vi "PvgeneratorOP500.vi"(8 "errin":errorcluster, 9 "BDD":T1, 10 "network":path, 11 "path in":path) -> (0 "sortie d'erreur":errorcluster caption="errout", 1 "network out":path, 2 "tout bon":bool, 3 "Chaîne":string)   [LabVIEW 2020]
uses:
  VG/IS30%.vi
  VG/PN.vi
panel:
  out "PDU+":string
  out "PDU-":string
  out "Tab1":string[][](array[string])
  out "nombre de remplacements":i32
  # "16/10/2023_08:15:59"
  # "2023-10-04 15:58:32"
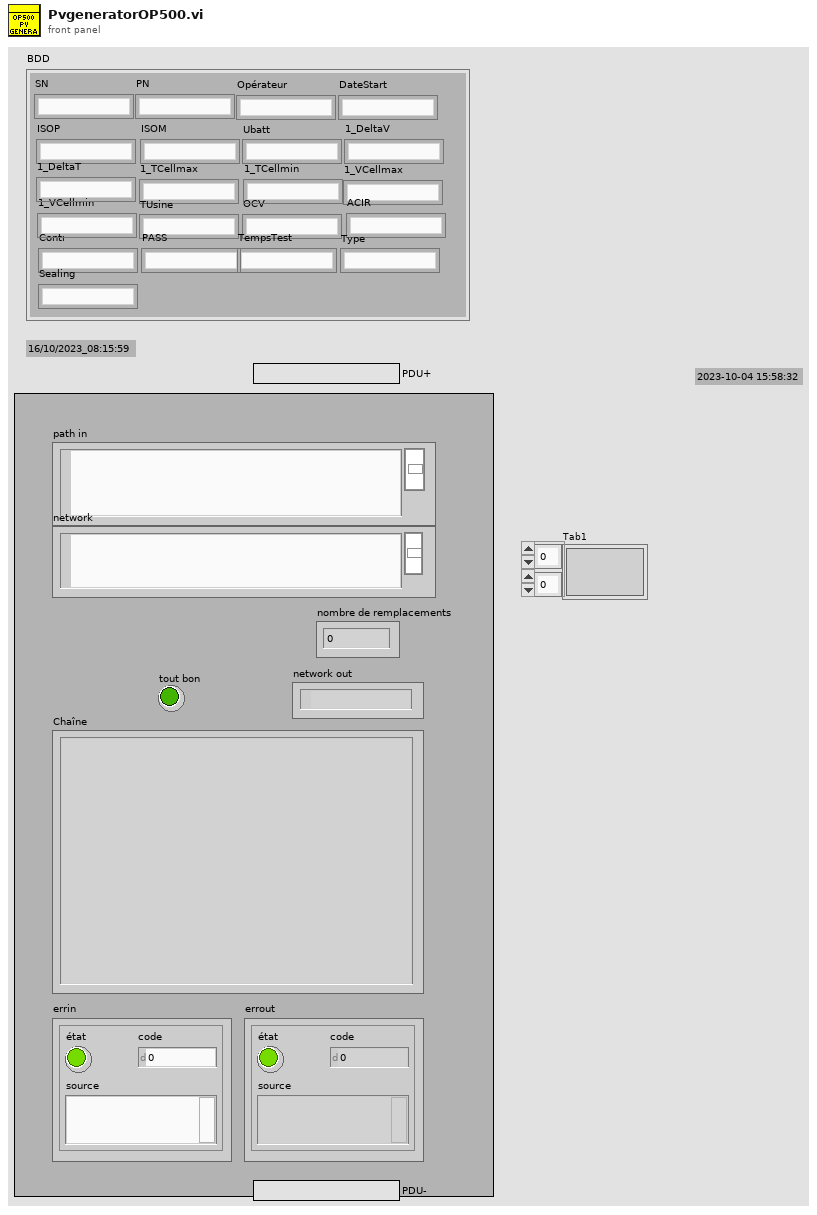
[diagram p1: front panel]
types:
  T1 = cluster{"SN":string, "PN":string, "Opérateur":string, "DateStart":string, "ISOP":string, "ISOM":string, "Ubatt":string, "1_DeltaV":string, "1_DeltaT":string, "1_TCellmax":string, "1_TCellmin":string, "1_VCellmax":string, "1_VCellmin":string, "TUsine":string, "OCV":string, "ACIR":string, "Conti":string, "PASS":string, "TempsTest":string, "Type":string, "Sealing":string}
  T2 = enum16{"open", "replace", "create", "open or create", "replace or create", "replace or create with confirmation"}
  T3 = cluster{string, string, string, string, string, string, string, string, string, string}
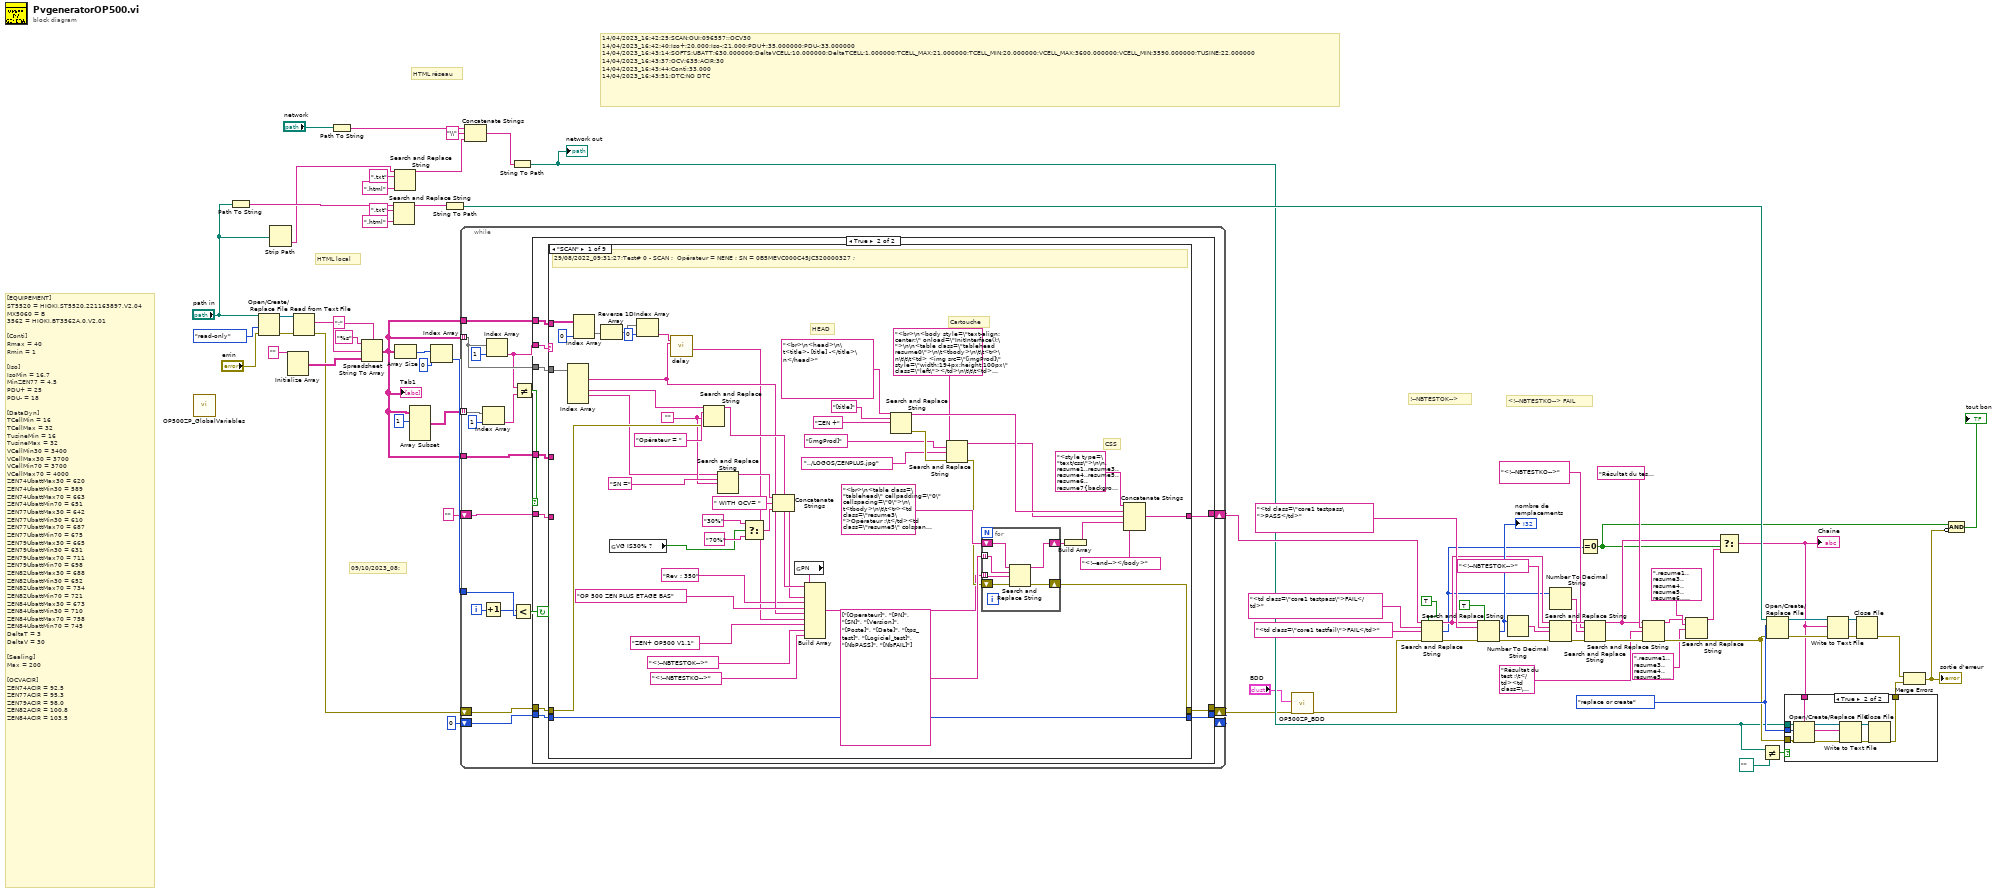
[diagram p0: block diagram]
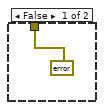
[diagram p2: hidden frame]
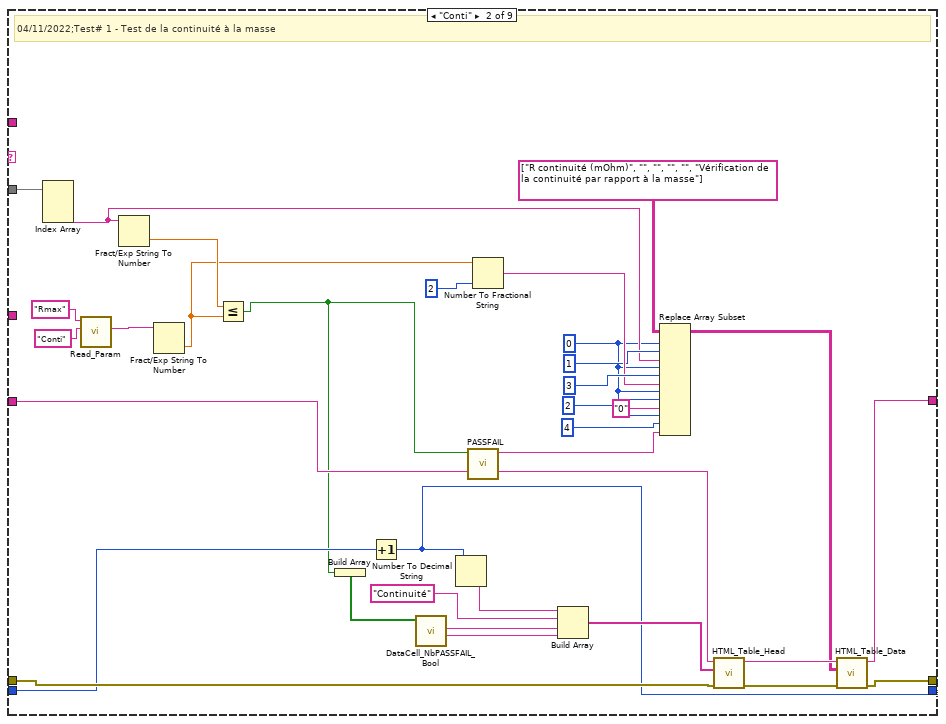
[diagram p4: hidden frame]
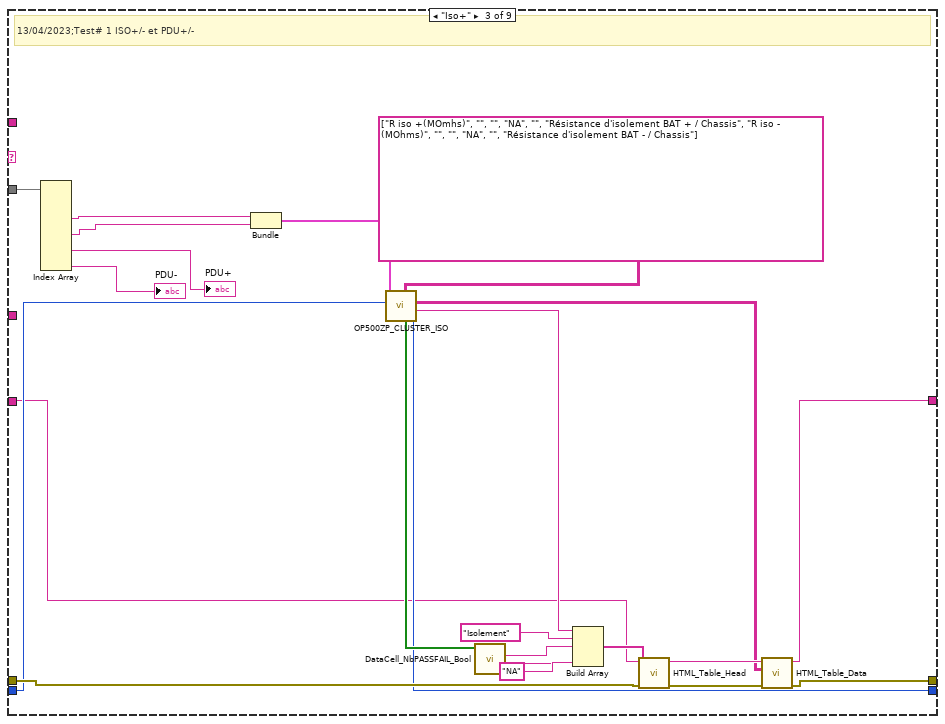
[diagram p5: hidden frame]
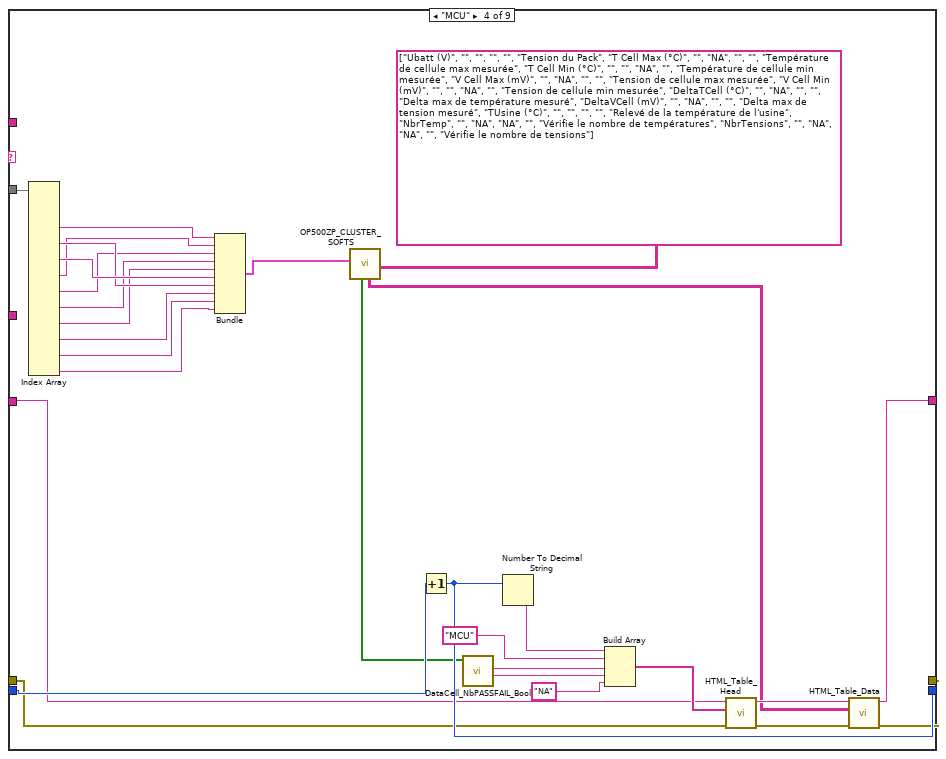
[diagram p6: hidden frame]
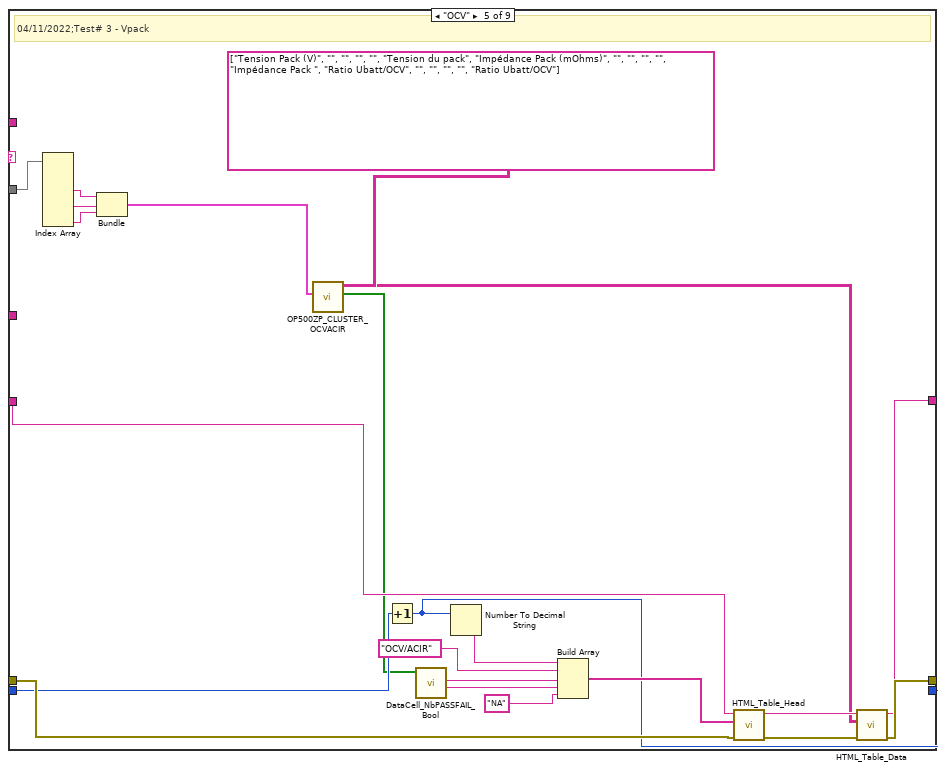
[diagram p7: hidden frame]
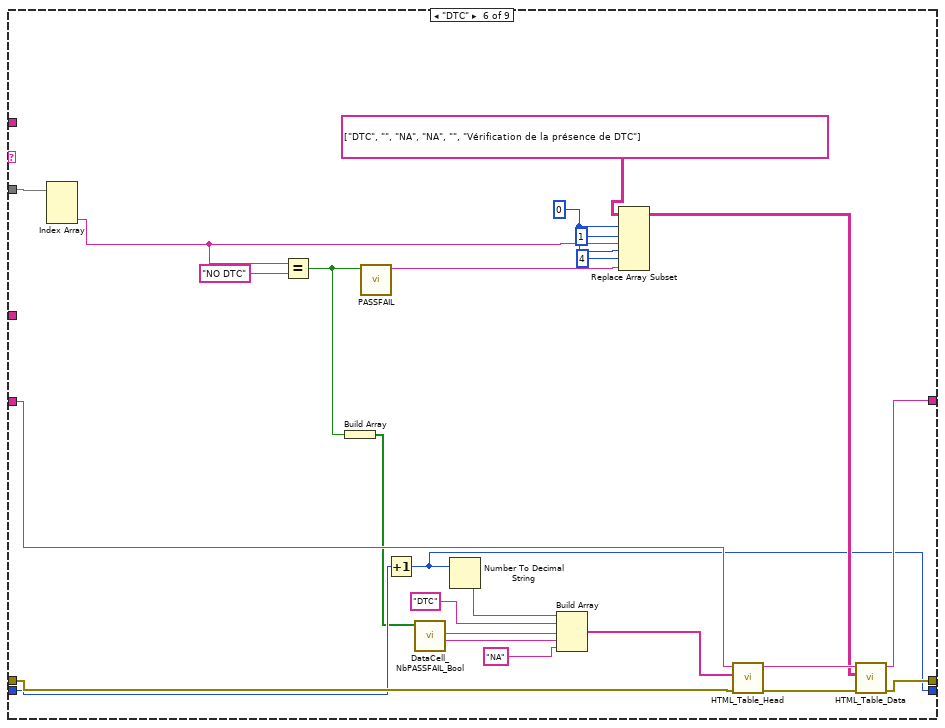
[diagram p8: hidden frame]
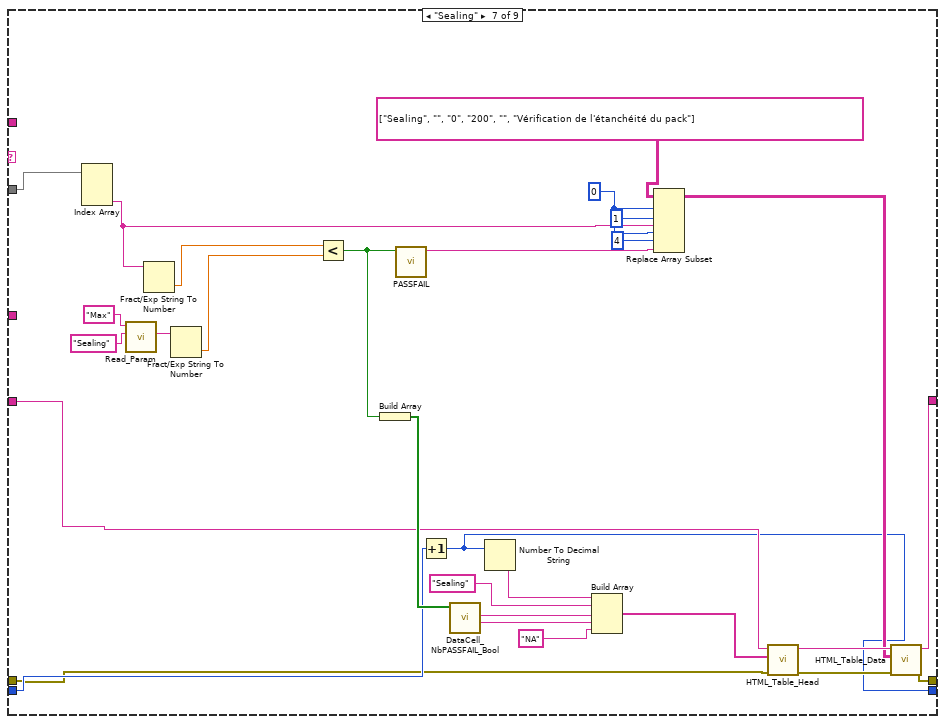
[diagram p9: hidden frame]
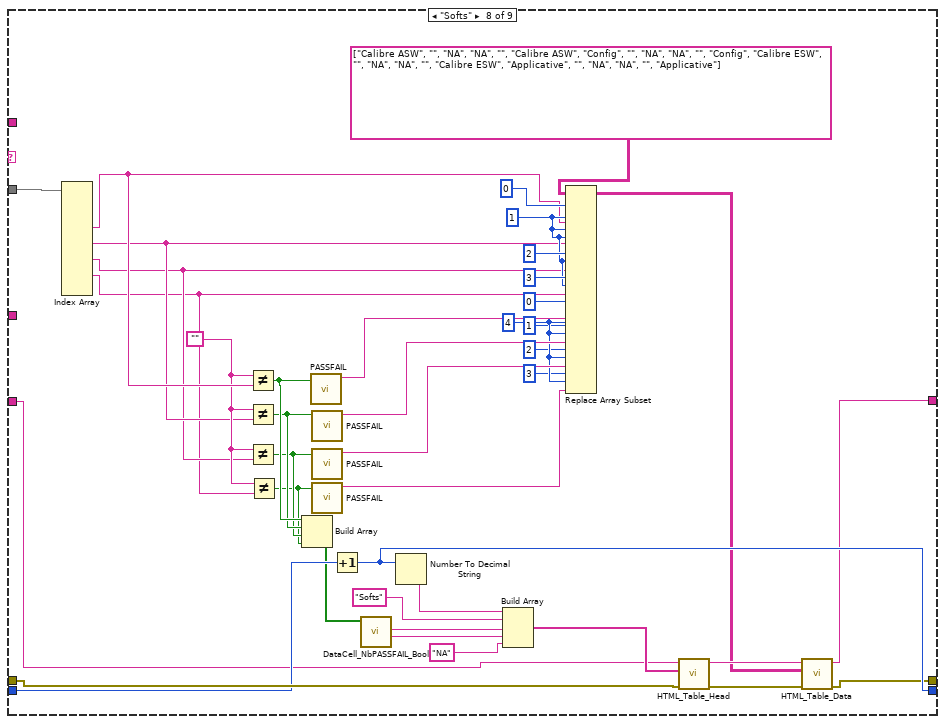
[diagram p10: hidden frame]
diagram:
  w36 = T2."replace or create" ("opération (0 : open)")
  # "09/10/2023_08:"
  # "HTML réseau"
  # "HTML local"
  # "14/04/2023_16:42:25;SCAN;OUI;096557;;OCV30\n14/04/2023_16:42:40;Iso+;20,000;Iso-;21,000;PDU+;35,000000;PDU-;33,000000\n14/04/2023_16:43:14;SOFTS;UBATT;630,000000;DeltaVCELL;10,000000;DeltaTCELL;1,000000;TCELL_MAX;21,000000;TCELL_MIN;20,000000;VCELL_MAX;3600,000000;VCELL_MIN;3590,000000;TUSINE;22,000000\n14/04/2023_16:43:37;OCV;635;ACIR;30\n14/04/2023_16:43:44;Conti;33,000\n14/04/2023_16:43:51;DTC;NO DTC"
  # "[EQUIPEMENT]\nST5520 = HIOKI,ST5520,221163897,V2.04\t\nMX5060 = B\n3562 = HIOKI,BT3562A,0,V2.01\n\n[Conti]\nRmax = 40\nRmin = 1\n\n[Iso]\nIsoMin = 16.7\nMinZEN77 = 4.5\nPDU+ = 25\nPDU- = 18\n\n[DataDyn]\nTCellMin = 16\nTCellMax = 32\nTusineMin = 16\nTusineMax = 32\nVCellMin30 = 3400\nVCellMax30 = 3700\nVCellMin70 = 3700\nVCellMax70 = 4000\nZEN74UbattMax30 = 620\nZEN74UbattMin30 = 589\nZEN74UbattMax70 = 663\nZEN74UbattMin70 = 651\nZEN77UbattMax30 = 642\nZEN77UbattMin30 = 610\nZEN77UbattMax70 = 687\nZEN77UbattMin70 = 675\nZEN79UbattMax30 = 665\nZEN79UbattMin30 = 631\nZEN79UbattMax70 = 711\nZEN79UbattMin70 = 698\nZEN82UbattMax30 = 688\nZEN82UbattMin30 = 652\nZEN82UbattMax70 = 734\nZEN82UbattMin70 = 721\nZEN84UbattMax30 = 673\nZEN84UbattMin30 = 710\nZEN84UbattMax70 = 758\nZEN84UbattMin70 = 745\nDeltaT = 3\nDeltaV = 30\n\n[Sealing]\nMax = 200\n\n[OCVACIR]\nZEN74ACIR = 92.5\nZEN77ACIR = 95.3\nZEN79ACIR = 98.0\nZEN82ACIR = 100.8\nZEN84ACIR = 103.5"
  # "<!--NBTESTKO--> FAIL"
  # "!--NBTESTOK-->"
  n1 = call "OP500ZP_GlobalVariables.vi"() -> ()  [unwired: 12 in]
  n2 = Path To String(path="path in") -> (string=w57:string)
  n3 = Open/Create/Replace File(file path (use dialog)="path in", error in="errin", access (0:read/write)=enum16{"read/write", "read-only", "write-only"}."read-only" ("accès (0 : read/write)")) -> (refnum out=w58:refnum<file>, error out=w74:errorcluster)  [unwired: 3 in, 1 out]
  n4 = Strip Path(path="path in") -> (name=w17:string)  [unwired: 1 out]
  n5 = Initialize Array("") -> (w72:string[][])  [unwired: 2 in]
  n6 = Read from Text File(file (use dialog)=w58, error in=w74) -> (text=w70:string, error out=w4:errorcluster)  [unwired: 2 in, 2 out]
  n7 = Path To String(path="network") -> (string=w16:string)
  n8 = Spreadsheet String To Array(delimiter (Tab)=";" ("séparateur (Tabulation)"), format string="%s" ("chaîne de format"), spreadsheet string=w70, array type (2D Dbl)=w72) -> (array=w7:string[][])
  "Tab1" <- w7
  n9 = Search and Replace String(input string=w57, search string=".txt" ("chaîne recherchée"), replace string=".html" ("chaîne de remplacement (\"\")")) -> (result string=w54:string)  [unwired: 5 in, 3 out]
  n10 = Search and Replace String(input string=w17, search string=".txt" ("chaîne recherchée"), replace string=".html" ("chaîne de remplacement (\"\")")) -> (result string=w14:string)  [unwired: 5 in, 3 out]
  n11 = Array Size(array=w7) -> (size(s)=w68:i32[])
  n12 = Array Subset(array=w7, index (row)=1 ("indice")) -> (w5:string[][])  [unwired: 3 in]
  n13 = Index Array(array=w68, index=0 ("indice")) -> (element=w66:i32)
  n14 = String To Path(string=w54) -> (path=w53:path)
  n15 = while {
    tunnel: w66 -> [w93]
    tunnel: w7 -> [w90] mode=indexing
    shift-right: [w89] -> w1
    shift-left: w4 -> [w88]
    shift-right: [w82] -> w52
    shift-left: "" -> [w87]
    shift-right: [w85] -> _
    shift-left: 0 -> [w86]
    tunnel: w7 -> [w84]
    tunnel: w7 -> [w81]
    tunnel: w5 -> [w79] mode=indexing
    i -> [w94]
    stop <- w92 continue-if-true
    n16 = Index Array(array=w79, index=1 ("indice")) -> (element=w78:string)
    n17 = Increment(x=w94) -> (x+1=w83:i32)
    n18 = Index Array(array=w90, index=1 ("indice")) -> (element=w77:string)
    n19 = Less?(x=w83, y=w93) -> (x < y?=w92:bool)
    n20 = Not Equal?(x=w77, y=w78) -> (x != y?=w76:bool)
    n21 = case shown="True" w76 {
      tunnel: w90 -> [_ w107]
      tunnel: [w96 w106] -> w89
      tunnel: w88 -> [w96 w105]
      tunnel: w87 -> [w97 w104]
      tunnel: w86 -> [w95 w103]
      tunnel: [w95 w102] -> w85
      tunnel: w84 -> [_ w101]
      tunnel: [w97 w100] -> w82
      tunnel: w77 -> [_ w99]
      tunnel: w81 -> [_ w98]
      frame False {
      }
      frame True {
        n22 = case shown="\"SCAN\"" w99 {
          tunnel: w105 -> [w154 w188 w211 w235 w261 w286 w305 w335 w366]
          tunnel: w107 -> [w156 w189 w212 w247 w262 w279 w307 w363 _]
          tunnel: [w133 w187 w210 w233 w260 w285 w302 w327 w366] -> w106
          tunnel: w104 -> [_ w186 w202 w232 w259 w280 w304 w324 w364]
          tunnel: w103 -> [w132 w185 w209 w239 w258 w284 w306 w334 w365]
          tunnel: [w132 w184 w203 w238 w257 w270 w301 w333 w365] -> w102
          tunnel: w101 -> [_ _ _ _ _ _ _ _ _]
          tunnel: [w131 w183 w208 w237 w256 w281 w303 w326 w364] -> w100
          tunnel: w98 -> [w110 _ _ _ _ _ _ _ _]
          frame "SCAN" {
            w127 = ""
            # "Cartouche"
            # "HEAD"
            # "CSS"
            # "29/08/2022_09:31:27;Test# 0 - SCAN ;  Opérateur = NENE ; SN = 0B5MEVC000C45JC320000327 ;"
            n23 = Index Array(array=w156) -> (element #1=w125:string, element #3=w130:string, element #4=w126:string)  [unwired: 5 in, 2 out]
            n24 = Index Array(array=w110, index (col)=0 ("disabled index (col)")) -> (element=w113:string[])  [unwired: 1 in]
            n25 = Reverse 1D Array(array=w113) -> (reversed array=w112:string[])
            n26 = global read "IS30%.vi" "VG IS30% ?"() -> (w117:bool)
            n27 = Index Array(array=w112, index=0) -> (element=w109:string)
            n28 = call "delay.vi"("String"=w125, "String 2"=w109) -> ("Delay calculé"=w108:string)  [unwired: 9 in]
            n29 = Search and Replace String(input string=w130, search string="Opérateur = " ("chaîne recherchée"), replace string=w127, error in=w154) -> (result string=w129:string)  [unwired: 4 in, 3 out]
            n30 = Search and Replace String(input string=w126, search string="SN =" ("chaîne recherchée"), replace string=w127) -> (result string=w123:string)  [unwired: 5 in, 3 out]
            n31 = Select(t="30%" ("y"), s=w117, f="70%" ("y")) -> (s? t:f=w120:string)
            n32 = Concatenate Strings(w123, " WITH OCV= " ("chaîne"), w120) -> (w122:string)
            n33 = global read "PN.vi" "PN"() -> (w116:string)
            n34 = Build Array(w129, w116, w122, "Rev : 350" ("élément"), "OP 500 ZEN PLUS ETAGE BAS" ("chaîne"), w125, w108, "ZEN+ OP500 V1.1" ("chaîne"), "<!--NBTESTOK-->" ("chaîne"), "<!--NBTESTKO-->" ("chaîne")) -> (w134:string[])
            n35 = Search and Replace String(input string="<br>\n<head>\n\t<title>- [title] -</title>\n</head>", search string="[title]" ("chaîne recherchée"), replace string="ZEN +" ("Title")) -> (result string=w150:string, error out=w149:errorcluster)  [unwired: 5 in, 2 out]
            n36 = Search and Replace String(input string="<br>\n<body style=\"text-align: center;\" onload=\"InitInterface();\">\n\n<table class=\"tablehead resume0\">\n\t<tbody>\n\t\t<tr>\n\t\t\t<td> <img src=\"[imgProd]\" style=\"width:194px;height:100px\" class=\"left\"></td>\n\t\t\t<td> <div class=\"center\">PROCES VERBAL DE TEST AUTOMATIQUE</div><div class=\"center\">Zen Plus OP 500</div><br class=\"center\"><div class=\"center\">Forseepower</div></td>\n\t\t\t<td> <img src=\"../LOGOS/LOGO FORSEE.png\" style=\"width:194px\"  class=\"right\"></td>\n\t\t</tr>\n\t</tbody>\n</table>", search string="[imgProd]", replace string="../LOGOS/ZENPLUS.jpg" ("imgProd"), error in=w149) -> (result string=w147:string, error out=w144:errorcluster)  [unwired: 4 in, 2 out]
            n37 = for {
              shift-right: [w161] -> w143
              shift-left: "<br>\n<table class=\"tablehead\" cellpadding=\"0\" cellspacing=\"0\">\n\t<tbody>\n\t\t<tr><td class=\"resume3\">Opérateur :\t</td><td class=\"resume5\" colspan=\"3\">[Operateur]</td></tr>\n\t\t<tr><td class=\"resume3\">PN : </td><td class=\"resume5\" colspan=\"3\">[PN]</td></tr>\n\t\t<tr><td class=\"resume3\">SN : </td><td class=\"resume5\" colspan=\"3\">[SN]</td></tr>\n\t\t<tr><td class=\"resume3\">Version : </td><td class=\"resume5\" colspan=\"3\">[Version]</td></tr>\n\t\t<tr><td class=\"resume3\">Poste : </td><td class=\"resume5\" colspan=\"3\">[Poste]</td></tr>\t\t\n\t\t<tr><td class=\"resume3\">Date du test : </td><td class=\"resume5\" colspan=\"3\">[Date]</td></tr>\n\t\t<tr><td class=\"resume3\">Temps de test : </td><td class=\"resume5\" colspan=\"3\">[tps_test]</td></tr>\n\t\t<tr><td class=\"resume3\">Logiciel de test :\t</td><td class=\"resume5\" colspan=\"3\">[Logiciel_test]</td></tr>\n\t\t<tr><td class=\"resume3\">Résultat du test :\t</td><td class=\"resume5\" colspan=\"3\"><div><span style=\"float:left\" id=\"result\"><font size = \"5pt\" color=\"green\"><b>CONFORME</b></font><b><font size = \"5pt\"> ( </font><font size = \"5pt\" color=\"green\">[NbPASS] PASS </font>  <font size = \"5pt\"> / </font><font size = \"5pt\" color=\"red\">[NbFAIL] FAIL</font> <font size = \"5pt\"> ) </font></b></span></div></td></tr>\n\t</tbody>\n</table>" -> [w162]
              tunnel: string[] ["[Operateur]", "[PN]", "[SN]", "[Version]", "[Poste]", "[Date]", "[tps_test]", "[Logiciel_test]", "[NbPASS]", "[NbFAIL]"] -> [w158] mode=indexing
              tunnel: w134 -> [w157] mode=indexing
              shift-right: [w159] -> w133
              shift-left: w144 -> [w160]
              n38 = Search and Replace String(input string=w162, search string=w158, replace string=w157, error in=w160) -> (result string=w161:string, error out=w159:errorcluster)  [unwired: 4 in, 2 out]
            }
            n39 = Build Array(w143) -> (w142:string[])
            n40 = Concatenate Strings("<style type=\"text/css\">\n\n.resume1,.resume3,.resume4,.resume5,.resume6,.resume7{background-color:#e6feef;padding:7px;border:1px solid black;}\n.resume0{border:1px solid black;background-color:#e6feef;font-weight: bold;padding:0px;text-align: center;}\n.resume1{width:350px;text-align:right;font-weight:bold;}\n.resume3{width:350px;text-align:right;border-top:0px solid black;font-weight:bold;}\n.resume4{border-left:0px solid black;width:290px;}\n.resume5{width:290px;border-left:0px solid black;border-top:0px solid black;}\n.resume6{border-left:0px solid black;width:60px;}\n.resume7{border-left:0px solid black;border-top:0px solid black;width:60px;}\n.title1{text-align: left;background-color:#e6f4fe;padding:10px;border:1px solid #101010;}\n.title2{width: 30px;text-align: center;background-color:#e6f4fe;padding:1px;border:1px solid #101010;border-left:0px solid black;font-weight: bold;}\n.title2 a:link{text-decoration:none;}\n.entete0,.entete1,.entete2,.time2{text-align: center;background-color:#feeec9;padding:7px;border:1px solid black;font-weight: bold;}\n.entete0{width:45px;border-right:0px solid black;}\n.entete1{width:505px;}\n.entete2{width:95px;border-right:0px solid black;}\n.time2{border-left:0px solid black;width:145px;font-size:11px;}\n.core0,.core1,.core2,.core3,.core4,.time{text-align: center;background-color:#fafed3;padding:7px;border:1px solid black;}\n.core0, .core1,.core3,.core4{width:95px;border-top:0px solid black;border-right:0px solid black;}\n.core0{width:45px;}\n.core2{border-top:0px solid black;width:505px;}\n.core3{width:200px;}\n.core4{width:300px;}\n.time{width:145px;border-top:0px solid black;border-left:0px solid black;font-size:11px;}\n.false .core0,.false .core1,.false .core2,.false .core3,.false .core4,.false .time{background-color:#f4f4f4;}\n.false .entete0,.false .entete1,.false .entete2,.false .time2{background-color:#dadada;}\n.false .title1,.false .title2,.false .resultentete .testpass,.false .resultentete .testfail,.false .resultentete .testtime{background-color:#c5cac9;color: blue;}\n.false .title2 a:link{text-decoration:none;color: blue;}\n.comment1,.comment2,.time3{width: 890px;background-color:#e9e8e9;padding:7px;border:1px solid black;border-top:0px solid black;text-align:left;}\n.comment2{border-right:0px solid black;width: 45px;text-align: center;}\n.time3{width: 145px;border-left:0px solid black;font-size:11px;}\n.fixe1{background: -moz-linear-gradient(center top , #101010 10%, #555555 80%) repeat scroll 0 0 transparent;background: -webkit-gradient(linear, left top, left bottom, from(#101010), to(#555555));border:2px solid orange;position : fixed;margin-top:20px;display:none;overflow-y:scroll;max-height:350px;text-shadow: 0px 0px 0 #333333;text-align:left;font-size:10px;padding:10px;margin-left:-162px;border-radius: 15px 15px 15px 15px;}\n.menufixe, .menufixelock{background: -moz-linear-gradient(center top , #101010 80%, transparent 20%) repeat scroll 0 0 transparent;background: -webkit-gradient(linear, left top, left bottom, from(#101010), color-stop(0.65, #101010), to(transparent)) repeat scroll 0 0 transparent;margin: -52px 0px 0px -9px;width:100%;position:fixed;height:55px;-moz-transition: margin 1s;-webkit-transition: margin 1s;}\n.menufixelock, .menufixe:hover{margin: -9px 0px 0px -9px;}\n.lockmenu, .separation,.separationmenu{text-align:center;background: -moz-linear-gradient(center top , #555555 10%, #111111 80%) repeat scroll 0 0 transparent;background: -webkit-gradient(linear, left top, left bottom, from(#555555), to(#111111));border: 1px solid white;border-radius: 10px 10px 10px 10px;box-shadow: 0 -1px 1px #555555 inset;color: #999999;font-weight: bold;width: 100px;padding: 2px;text-decoration: none;}\n.tablehead{width: 1000px;font-family: Verdana;font-size: 12px;margin-left: auto;margin-right: auto;}\n.tablenull{font-family: Verdana;font-size: 11px;margin-left: auto;margin-right: auto;}\n.separationmenu:hover div{display: inline;}\n.lockmenu:hover, .separation:hover,.separationmenu:hover{border: 1px solid orange;cursor:pointer;}\n.lockmenu:hover{border: 1px solid red;cursor:pointer;}\n.separationright{padding:10px;}\ndiv a:link{text-decoration:none;color:#cbcbcb;}\ndiv a:hover{text-decoration:underline;color:#cbcbcb;}\nspan a:link{text-decoration:none;color:#cbcbcb;}\nspan a:hover{text-decoration:none;color:#cbcbcb;}\n.false{color: blue;}\n.testpass{color: green;font-weight: bold;}\n.testfail{color: red;font-weight: bold;}\n.testtime{color: blue;font-weight: bold;}\n.resultentete{font-weight: bold;font-size: 11px;min-width: 200px;text-align:right;}\n.infohard{border: 1px solid black;background-color: white;text-align: center;width: 16px;height: 16px;border-radius: 5px;font-weight: bold;box-shadow: 0 -1px 2px #555555 inset;}\n.infohard:hover{background-color:#feeec9;cursor:pointer;}\n.footerhard{padding-top:30px;}\n.confighard{font-size:10px;width:110px;}\n.circlemain{margin-left:auto;margin-right:auto;}\n.circletext,.circleform{padding-top: 3px;text-align:center;font-size: 10px;width:200px;}\n.circleform{padding-bottom: 3px;padding-top: 1px;}\n.circle{border: 1px solid black;border-collapse: collapse;border-radius: 15px;box-shadow: 1px 1px 0 #505050;height: 15px;width: 15px;display:inline-block;}\n.bookmarkon, .bookmarkoff{background-color: yellow;border: 1px solid black;border-collapse: collapse;border-radius: 10px 10px 10px 10px;box-shadow: 1px 1px 0 #505050;height: 12px;width: 12px;position: absolute;margin-left:22px;cursor: help;}\n.bookmarkoff{background-color: transparent;border: 1px solid #CECECE;box-shadow: none;cursor: copy;}\n.false .bookmarkoff{background-color: transparent;border: 1px solid #E6E1E1;box-shadow: none;cursor: copy;}\n.bookmarkmaster{height: 15px;margin-right: 12px;width: 60px;}\n.bookmarkmaster:hover .bookmarkprev,.bookmarkmaster:hover .bookmarksuiv{display:block;}\n.bookmarkprev, .bookmarksuiv {cursor: pointer;font-size: 25px;font-weight: bold;margin-top: -10px;position: absolute;display:none;}\n.bookmarkprev{margin-left: 2px;}\n.bookmarksuiv{margin-left: 43px;}\n.plus, .moins{background-color: #F4F4F4;border: 1px solid #848484;border-radius: 20px;color: #848484;font-family: arial;font-size: 16px;font-weight: bold;height: 20px;margin-left: 4px;text-align: center;width: 20px;}\n.moins{font-size: 15px;}\n.plus:hover, .moins:hover{background-color: #DADADA;border: 1px solid black;color: black;cursor:pointer;}\n.backtothetop {position: fixed; right: 50%; margin-right: -555px; bottom: 10px; font-size: 35px; font-weight: bold; border: 1px solid #7D7B91; width: 40px; height: 40px; line-height:52px; text-align: center;border-radius: 8px; opacity: 0.25; background-color: #F5F5F5; color:#7D7B91;}\n.backtothetop:hover {opacity: 1; cursor:pointer;}\n.libversion {font-size: 8px;font-weight: normal;padding-right: 10px;text-align: right;}\n.lockmenu {width: 18px;font-size: 12px;}\n.left {display: block; margin-left: 1px;margin-right: auto;}\n.right {display: block; margin-right: 1px;margin-left: auto;}\n.center {display: block; margin-left: auto;margin-right: auto;}\n\n</style>", w150, w147, w142, "<!--end--></body>") -> (w131:string)
          }
          frame "Conti" {
            w171 = 0 ("index (row)")
            # "04/11/2022;Test# 1 - Test de la continuité à la masse"
            n41 = Index Array(array=w189) -> (element #3=w174:string)  [unwired: 3 in, 2 out]
            n42 = call <userlib>:"Read_Param.vi"("section"="Conti", "key"="Rmax") -> ("str"=w166:string)  [unwired: 5 in, 4 out]
            n43 = Fract/Exp String To Number(string=w174) -> (number=w169:dbl)  [unwired: 3 in, 1 out]
            n44 = Fract/Exp String To Number(string=w166) -> (number=w163:dbl)  [unwired: 3 in, 1 out]
            n45 = Less Or Equal?(x=w169, y=w163) -> (x <= y?=w168:bool)
            n46 = Build Array(w168) -> (w181:bool[])
            n47 = Increment(x=w185) -> (x+1=w184:i32)
            n48 = call <userlib>:"DataCell_NbPASSFAIL_Bool.vi"("Tableau en entrée"=w181) -> ("Chaîne"=w179:string, "Chaîne 2"=w180:string)  [unwired: 8 in, 1 out]
            n49 = Number To Decimal String(number=w184) -> (decimal integer string=w191:string)  [unwired: 1 in]
            n50 = call <userlib>:"PASSFAIL.vi"("E"=w168) -> ("S"=w173:string)  [unwired: 10 in]
            n51 = Number To Fractional String(number=w163, precision (6)=i16 2) -> (F-format string=w177:string)  [unwired: 2 in]
            n52 = Build Array(w191, "Continuité" ("élément"), w180, w179) -> (w194:string[])
            n53 = Replace Array Subset(array=string[][] [["R continuité (mOhm)", "", "", "", "", "Vérification de la continuité par rapport à la masse"]] ("Tableau"), new element #1=w174, index (row) #1=w171, index (col) #1=1 ("disabled index (col)"), new element #2=w177, index (row) #2=w171, index (col) #2=3 ("disabled index (col)"), new element #3="0" ("nouvel élément/sous-tableau"), index (row) #3=w171, index (col) #3=2 ("disabled index (col)"), new element #4=w173, index (row) #4=w171, index (col) #4=4 ("disabled index (col)")) -> (w182:string[][])
            n54 = call "HTML_Table_Head.vi"("entrée d'erreur (pas d'erreur)"=w188, "Tableau"=w194, "chaîne en entrée"=w186) -> ("sortie d'erreur"=w193:errorcluster, "result string"=w192:string)  [unwired: 7 in]
            n55 = call "HTML_Table_Data.vi"("entrée d'erreur (pas d'erreur)"=w193, "Tableau"=w182, "chaîne en entrée"=w192) -> ("sortie d'erreur"=w187:errorcluster, "result string"=w183:string)  [unwired: 7 in]
          }
          frame "Iso+" {
            # "13/04/2023;Test# 1 ISO+/- et PDU+/-"
            n56 = Index Array(array=w212) -> (element #3=w201:string, element #5=w200:string, element #7=→"PDU+":string, element #9=→"PDU-":string)  [unwired: 9 in, 5 out]
            n57 = Bundle(w201, w200) -> (w197:cluster{string, string})  [unwired: 1 in]
            n58 = call "OP500ZP_CLUSTER_ISO.vi"("Tableau 3"=string[][] [["R iso +(MOmhs)", "", "", "NA", "", "Résistance d'isolement BAT + / Chassis"], ["R iso - (MOhms)", "", "", "NA", "", "Résistance d'isolement BAT - / Chassis"]] ("Tableau"), "Numérique en entrée"=w209, "MESURES ISO"=w197) -> ("Chaîne"=w215:string, "Tableau 2"=w207:string[][], "Numérique en sortie"=w203:i32, "Tableau"=w206:bool[])  [unwired: 5 in]
            n59 = call <userlib>:"DataCell_NbPASSFAIL_Bool.vi"("Tableau en entrée"=w206) -> ("Chaîne"=w204:string, "Chaîne 2"=w205:string)  [unwired: 8 in, 1 out]
            n60 = Build Array(w215, "Isolement" ("élément"), w205, w204, "NA" ("élément")) -> (w218:string[])
            n61 = call "HTML_Table_Head.vi"("entrée d'erreur (pas d'erreur)"=w211, "Tableau"=w218, "chaîne en entrée"=w202) -> ("sortie d'erreur"=w217:errorcluster, "result string"=w216:string)  [unwired: 7 in]
            n62 = call "HTML_Table_Data.vi"("entrée d'erreur (pas d'erreur)"=w217, "Tableau"=w207, "chaîne en entrée"=w216) -> ("sortie d'erreur"=w210:errorcluster, "result string"=w208:string)  [unwired: 7 in]
          }
          frame "MCU" {
            n63 = Index Array(array=w247) -> (element #4=w231:string, element #6=w229:string, element #8=w230:string, element #10=w226:string, element #12=w225:string, element #14=w228:string, element #16=w227:string, element #18=w222:string, element #20=w220:string, element #22=w219:string)  [unwired: 22 in, 12 out]
            n64 = Bundle(w231, w226, w225, w228, w227, w230, w229, w222, w220, w219) -> (w221:T3)  [unwired: 1 in]
            n65 = call "OP500ZP_CLUSTER_SOFTS.vi"("MESURES"=w221, "EmptyTab"=string[][] [["Ubatt (V)", "", "", "", "", "Tension du Pack"], ["T Cell Max (°C)", "", "NA", "", "", "Température de cellule max mesurée"], ["T Cell Min (°C)", "", "", "NA", "", "Température de cellule min mesurée"], ["V Cell Max (mV)", "", "NA", "", "", "Tension de cellule max mesurée"], ["V Cell Min (mV)", "", "", "NA", "", "Tension de cellule min mesurée"], ["DeltaTCell (°C)", "", "NA", "", "", "Delta max de température mesuré"], ["DeltaVCell (mV)", "", "NA", "", "", "Delta max de tension mesuré"], ["TUsine (°C)", "", "", "", "", "Relevé de la température de l'usine"], ["NbrTemp", "", "NA", "NA", "", "Vérifie le nombre de températures"], ["NbrTensions", "", "NA", "NA", "", "Vérifie le nombre de tensions"]] ("Tableau")) -> ("Tab1"=w224:string[][], "PASS/FAIL"=w223:bool[])  [unwired: 8 in]
            n66 = Increment(x=w239) -> (x+1=w238:i32)
            n67 = call <userlib>:"DataCell_NbPASSFAIL_Bool.vi"("Tableau en entrée"=w223) -> ("Chaîne"=w240:string, "Chaîne 2"=w241:string)  [unwired: 8 in, 1 out]
            n68 = Number To Decimal String(number=w238) -> (decimal integer string=w244:string)  [unwired: 1 in]
            n69 = Build Array(w244, "MCU" ("élément"), w241, w240, "NA" ("élément")) -> (w246:string[])
            n70 = call "HTML_Table_Head.vi"("entrée d'erreur (pas d'erreur)"=w235, "Tableau"=w246, "chaîne en entrée"=w232) -> ("sortie d'erreur"=w234:errorcluster, "result string"=w245:string)  [unwired: 7 in]
            n71 = call "HTML_Table_Data.vi"("entrée d'erreur (pas d'erreur)"=w234, "Tableau"=w224, "chaîne en entrée"=w245) -> ("sortie d'erreur"=w233:errorcluster, "result string"=w237:string)  [unwired: 7 in]
          }
          frame "OCV" {
            # "04/11/2022;Test# 3 - Vpack"
            n72 = Index Array(array=w262) -> (element #3=w251:string, element #5=w250:string, element #7=w248:string)  [unwired: 7 in, 4 out]
            n73 = Bundle(w251, w250, w248) -> (w249:cluster{string, string, string})  [unwired: 1 in]
            n74 = call "OP500ZP_CLUSTER_OCVACIR.vi"("MESURES_OCVACIR"=w249, "Tableau 3"=string[][] [["Tension Pack (V)", "", "", "", "", "Tension du pack"], ["Impédance Pack (mOhms)", "", "", "", "", "Impédance Pack "], ["Ratio Ubatt/OCV", "", "", "", "", "Ratio Ubatt/OCV"]] ("Tableau")) -> ("Tableau"=w254:bool[], "Tableau 2"=w255:string[][])  [unwired: 8 in]
            n75 = Increment(x=w258) -> (x+1=w257:i32)
            n76 = call <userlib>:"DataCell_NbPASSFAIL_Bool.vi"("Tableau en entrée"=w254) -> ("Chaîne"=w252:string, "Chaîne 2"=w253:string)  [unwired: 8 in, 1 out]
            n77 = Number To Decimal String(number=w257) -> (decimal integer string=w265:string)  [unwired: 1 in]
            n78 = Build Array(w265, "OCV/ACIR" ("élément"), w253, w252, "NA" ("élément")) -> (w268:string[])
            n79 = call "HTML_Table_Head.vi"("entrée d'erreur (pas d'erreur)"=w261, "Tableau"=w268, "chaîne en entrée"=w259) -> ("sortie d'erreur"=w267:errorcluster, "result string"=w266:string)  [unwired: 7 in]
            n80 = call "HTML_Table_Data.vi"("entrée d'erreur (pas d'erreur)"=w267, "Tableau"=w255, "chaîne en entrée"=w266) -> ("sortie d'erreur"=w260:errorcluster, "result string"=w256:string)  [unwired: 7 in]
          }
          frame "DTC" {
            w275 = 0 ("indice (ligne)")
            n81 = Index Array(array=w279) -> (element #3=w277:string)  [unwired: 3 in, 2 out]
            n82 = Equal?(x=w277, y="NO DTC") -> (x = y?=w272:bool)
            n83 = Build Array(w272) -> (w271:bool[])
            n84 = call <userlib>:"PASSFAIL.vi"("E"=w272) -> ("S"=w273:string)  [unwired: 10 in]
            n85 = Increment(x=w284) -> (x+1=w270:i32)
            n86 = call <userlib>:"DataCell_NbPASSFAIL_Bool.vi"("Tableau en entrée"=w271) -> ("Chaîne"=w287:string, "Chaîne 2"=w288:string)  [unwired: 8 in, 1 out]
            n87 = Number To Decimal String(number=w270) -> (decimal integer string=w291:string)  [unwired: 1 in]
            n88 = Build Array(w291, "DTC" ("élément"), w288, w287, "NA" ("élément")) -> (w294:string[])
            n89 = Replace Array Subset(array=string[][] [["DTC", "", "NA", "NA", "", "Vérification de la présence de DTC"]] ("Tableau"), new element #1=w277, index (row) #1=w275, index (col) #1=1 ("indice désactivé (col)"), new element #2=w273, index (row) #2=w275, index (col) #2=4 ("indice désactivé (col)")) -> (w282:string[][])
            n90 = call "HTML_Table_Head.vi"("entrée d'erreur (pas d'erreur)"=w286, "Tableau"=w294, "chaîne en entrée"=w280) -> ("sortie d'erreur"=w293:errorcluster, "result string"=w292:string)  [unwired: 7 in]
            n91 = call "HTML_Table_Data.vi"("entrée d'erreur (pas d'erreur)"=w293, "Tableau"=w282, "chaîne en entrée"=w292) -> ("sortie d'erreur"=w285:errorcluster, "result string"=w281:string)  [unwired: 7 in]
          }
          frame "Sealing" {
            w312 = 0 ("indice (ligne)")
            n92 = Index Array(array=w307) -> (element #3=w297:string)  [unwired: 3 in, 2 out]
            n93 = call <userlib>:"Read_Param.vi"("section"="Sealing", "key"="Max") -> ("str"=w300:string)  [unwired: 5 in, 4 out]
            n94 = Fract/Exp String To Number(string=w297) -> (number=w296:dbl)  [unwired: 3 in, 1 out]
            n95 = Fract/Exp String To Number(string=w300) -> (number=w295:dbl)  [unwired: 3 in, 1 out]
            n96 = Less?(x=w296, y=w295) -> (x < y?=w309:bool)
            n97 = Build Array(w309) -> (w308:bool[])
            n98 = call <userlib>:"PASSFAIL.vi"("E"=w309) -> ("S"=w310:string)  [unwired: 10 in]
            n99 = Increment(x=w306) -> (x+1=w301:i32)
            n100 = call <userlib>:"DataCell_NbPASSFAIL_Bool.vi"("Tableau en entrée"=w308) -> ("Chaîne"=w316:string, "Chaîne 2"=w317:string)  [unwired: 8 in, 1 out]
            n101 = Number To Decimal String(number=w301) -> (decimal integer string=w320:string)  [unwired: 1 in]
            n102 = Build Array(w320, "Sealing" ("élément"), w317, w316, "NA" ("élément")) -> (w323:string[])
            n103 = Replace Array Subset(array=string[][] [["Sealing", "", "0", "200", "", "Vérification de l'étanchéité du pack"]] ("Tableau"), new element #1=w297, index (row) #1=w312, index (col) #1=1 ("indice désactivé (col)"), new element #2=w310, index (row) #2=w312, index (col) #2=4 ("indice désactivé (col)")) -> (w314:string[][])
            n104 = call "HTML_Table_Head.vi"("entrée d'erreur (pas d'erreur)"=w305, "Tableau"=w323, "chaîne en entrée"=w304) -> ("sortie d'erreur"=w322:errorcluster, "result string"=w321:string)  [unwired: 7 in]
            n105 = call "HTML_Table_Data.vi"("entrée d'erreur (pas d'erreur)"=w322, "Tableau"=w314, "chaîne en entrée"=w321) -> ("sortie d'erreur"=w302:errorcluster, "result string"=w303:string)  [unwired: 7 in]
          }
          frame "Softs" {
            w347 = 4 ("indice désactivé (col)")
            w356 = ""
            w358 = 1 ("indice désactivé (col)")
            n106 = Index Array(array=w363) -> (element #4=w357:string, element #6=w355:string, element #8=w354:string, element #10=w353:string)  [unwired: 12 in, 8 out]
            n107 = Not Equal?(x=w356, y=w357) -> (x != y?=w332:bool)
            n108 = Not Equal?(x=w356, y=w355) -> (x != y?=w331:bool)
            n109 = Not Equal?(x=w356, y=w354) -> (x != y?=w330:bool)
            n110 = Not Equal?(x=w356, y=w353) -> (x != y?=w329:bool)
            n111 = Build Array(w332, w331, w330, w329) -> (w328:bool[])
            n112 = call <userlib>:"PASSFAIL.vi"("E"=w332) -> ("S"=w352:string)  [unwired: 10 in]
            n113 = call <userlib>:"PASSFAIL.vi"("E"=w331) -> ("S"=w351:string)  [unwired: 10 in]
            n114 = call <userlib>:"PASSFAIL.vi"("E"=w330) -> ("S"=w350:string)  [unwired: 10 in]
            n115 = call <userlib>:"PASSFAIL.vi"("E"=w329) -> ("S"=w349:string)  [unwired: 10 in]
            n116 = Increment(x=w334) -> (x+1=w333:i32)
            n117 = call <userlib>:"DataCell_NbPASSFAIL_Bool.vi"("Tableau en entrée"=w328) -> ("Chaîne"=w336:string, "Chaîne 2"=w337:string)  [unwired: 8 in, 1 out]
            n118 = Number To Decimal String(number=w333) -> (decimal integer string=w340:string)  [unwired: 1 in]
            n119 = Build Array(w340, "Softs" ("élément"), w337, w336, "NA" ("élément")) -> (w343:string[])
            n120 = Replace Array Subset(array=string[][] [["Calibre ASW", "", "NA", "NA", "", "Calibre ASW"], ["Config", "", "NA", "NA", "", "Config"], ["Calibre ESW", "", "NA", "NA", "", "Calibre ESW"], ["Applicative", "", "NA", "NA", "", "Applicative"]] ("Tableau"), new element #1=w357, index (row) #1=0 ("indice (ligne)"), index (col) #1=w358, new element #2=w355, index (row) #2=w358, index (col) #2=w358, new element #3=w354, index (row) #3=2 ("indice (ligne)"), index (col) #3=w358, new element #4=w353, index (row) #4=3 ("indice (ligne)"), index (col) #4=w358, new element #5=w352, index (row) #5=0 ("indice (ligne)"), index (col) #5=w347, new element #6=w351, index (row) #6=1 ("indice désactivé (ligne)"), index (col) #6=w347, new element #7=w350, index (row) #7=2 ("indice désactivé (ligne)"), index (col) #7=w347, new element #8=w349, index (row) #8=3 ("indice désactivé (ligne)"), index (col) #8=w347) -> (w325:string[][])
            n121 = call "HTML_Table_Head.vi"("entrée d'erreur (pas d'erreur)"=w335, "Tableau"=w343, "chaîne en entrée"=w324) -> ("sortie d'erreur"=w342:errorcluster, "result string"=w341:string)  [unwired: 7 in]
            n122 = call "HTML_Table_Data.vi"("entrée d'erreur (pas d'erreur)"=w342, "Tableau"=w325, "chaîne en entrée"=w341) -> ("sortie d'erreur"=w327:errorcluster, "result string"=w326:string)  [unwired: 7 in]
          }
          frame "NULL", Default {
            # "NULL"
          }
        }
      }
    }
  }
  n123 = Concatenate Strings(w16, "\\" ("chaîne"), w14) -> (w13:string)
  n124 = String To Path(string=w13) -> (path=w19:path)
  "network out" <- w19
  n125 = call "OP500ZP_BDD.vi"("errin"=w1, "DATA IN"="BDD") -> ("error out"=w3:errorcluster)  [unwired: 9 in]
  n126 = Search and Replace String(replace all?=TRUE ("tout remplacer ? (F)"), input string=w52, search string="<td class=\"core1 testpass\">FAIL</td>" ("chaîne recherchée"), replace string="<td class=\"core1 testfail\">FAIL</td>" ("chaîne de remplacement (\"\")"), error in=w3) -> (result string=w37:string, number of replacements=w32:i32, error out=w48:errorcluster)  [unwired: 3 in, 1 out]
  n127 = Search and Replace String(replace all?=TRUE ("tout remplacer ? (F)"), input string=w37, search string="<td class=\"core1 testpass\">PASS</td>" ("chaîne recherchée"), error in=w48) -> (number of replacements=w40:i32, error out=w44:errorcluster)  [unwired: 4 in, 2 out]
  "nombre de remplacements" <- w40
  n128 = Number To Decimal String(number=w40) -> (decimal integer string=w39:string)  [unwired: 1 in]
  n129 = Number To Decimal String(number=w32) -> (decimal integer string=w38:string)  [unwired: 1 in]
  n130 = Search and Replace String(input string=w37, search string="<!--NBTESTOK-->" ("chaîne recherchée"), replace string=w39, error in=w44) -> (result string=w45:string, error out=w43:errorcluster)  [unwired: 4 in, 2 out]
  n131 = Equal To 0?(x=w32) -> (x = 0?=w24:bool)
  n132 = Search and Replace String(input string=w45, search string="<!--NBTESTKO-->" ("chaîne recherchée"), replace string=w38, error in=w43) -> (result string=w27:string, error out=w31:errorcluster)  [unwired: 4 in, 2 out]
  n133 = Search and Replace String(input string=w27, search string="Résultat du test :\t</td><td class=\"resume5\" colspan=\"3\"><div><span style=\"float:left\" id=\"result\"><font size = \"5pt\" color=\"green\"><b>CONFORME</b>", replace string="Résultat du test :\t</td><td class=\"resume5\" colspan=\"3\"><div><span style=\"float:left\" id=\"result\"><font  size = \"5pt\" color=\"red\"><b>NON CONFORME</b>", error in=w31) -> (result string=w9:string, error out=w30:errorcluster)  [unwired: 4 in, 2 out]
  n134 = Search and Replace String(input string=w9, search string=".resume1,.resume3,.resume4,.resume5,.resume6,.resume7{background-color:#e6feef;padding:7px;border:1px solid black;}\n.resume0{border:1px solid black;background-color:#e6feef;font-weight: bold;padding:0px;text-align: center;}", replace string=".resume1,.resume3,.resume4,.resume5,.resume6,.resume7{background-color:#fdebd0;padding:7px;border:1px solid black;}\n.resume0{border:1px solid black;background-color:#fdebd0;font-weight: bold;padding:0px;text-align: center;}") -> (result string=w8:string)  [unwired: 5 in, 3 out]
  n135 = Select(t=w27, s=w24, f=w8) -> (s? t:f=w28:string)
  "Chaîne" <- w28
  n136 = Not Equal?(x=w19, y=path "") -> (x != y?=w21:bool)
  n137 = Open/Create/Replace File(file path (use dialog)=w53, error in=w30, operation (0:open)=w36) -> (refnum out=w59:refnum<file>, error out=w61:errorcluster)  [unwired: 3 in, 1 out]
  n138 = case shown="True" w21 {
    tunnel: w36 -> [_ w372]
    tunnel: w19 -> [_ w371]
    tunnel: w30 -> [_ w370]
    tunnel: w28 -> [_ w369]
    tunnel: [errorcluster {"status"=FALSE, "code"=0, "source"=""} ("error out") w368] -> w26
    frame False {
    }
    frame True {
      n139 = Open/Create/Replace File(file path (use dialog)=w371, error in=w370, operation (0:open)=w372) -> (refnum out=w373:refnum<file>, error out=w375:errorcluster)  [unwired: 3 in, 1 out]
      n140 = Write to Text File(file (use dialog)=w373, text=w369, error in=w375) -> (refnum out=w374:refnum<file>, error out=w376:errorcluster)  [unwired: 1 in, 1 out]
      n141 = Close File(refnum=w374, error in=w376) -> (error out=w368:errorcluster)  [unwired: 1 out]
    }
  }
  n142 = Write to Text File(file (use dialog)=w59, text=w28, error in=w61) -> (refnum out=w60:refnum<file>, error out=w62:errorcluster)  [unwired: 1 in, 1 out]
  n143 = Close File(refnum=w60, error in=w62) -> (error out=w25:errorcluster)  [unwired: 1 out]
  n144 = Merge Errors(w25, w26) -> (w23:errorcluster)
  "sortie d'erreur" <- w23
  n145 = Compound Arithmetic op=AND ("Opérateur arithmétique")(w24, invert w23) -> (→"tout bon":bool)
